vi "11_LAYOUT_COVID_19_KIT.vi"() -> ()   [LabVIEW 2019]
panel:
  in  "INT_TAB":bool
  in  "Tab Control":enum32{"Page 1", "Page 2"}(tab)
  in  "vi path":path
  in  "stop":bool
  # "LAYOUT --> TAB/SUB"
  # "SELECTOR TAB"
  # "(C) 2020"
  # "J.LUIS PÉREZ DEL VAL"
  # "GIF ANIMADO"
  # "KIT o CALENDARIO?..."
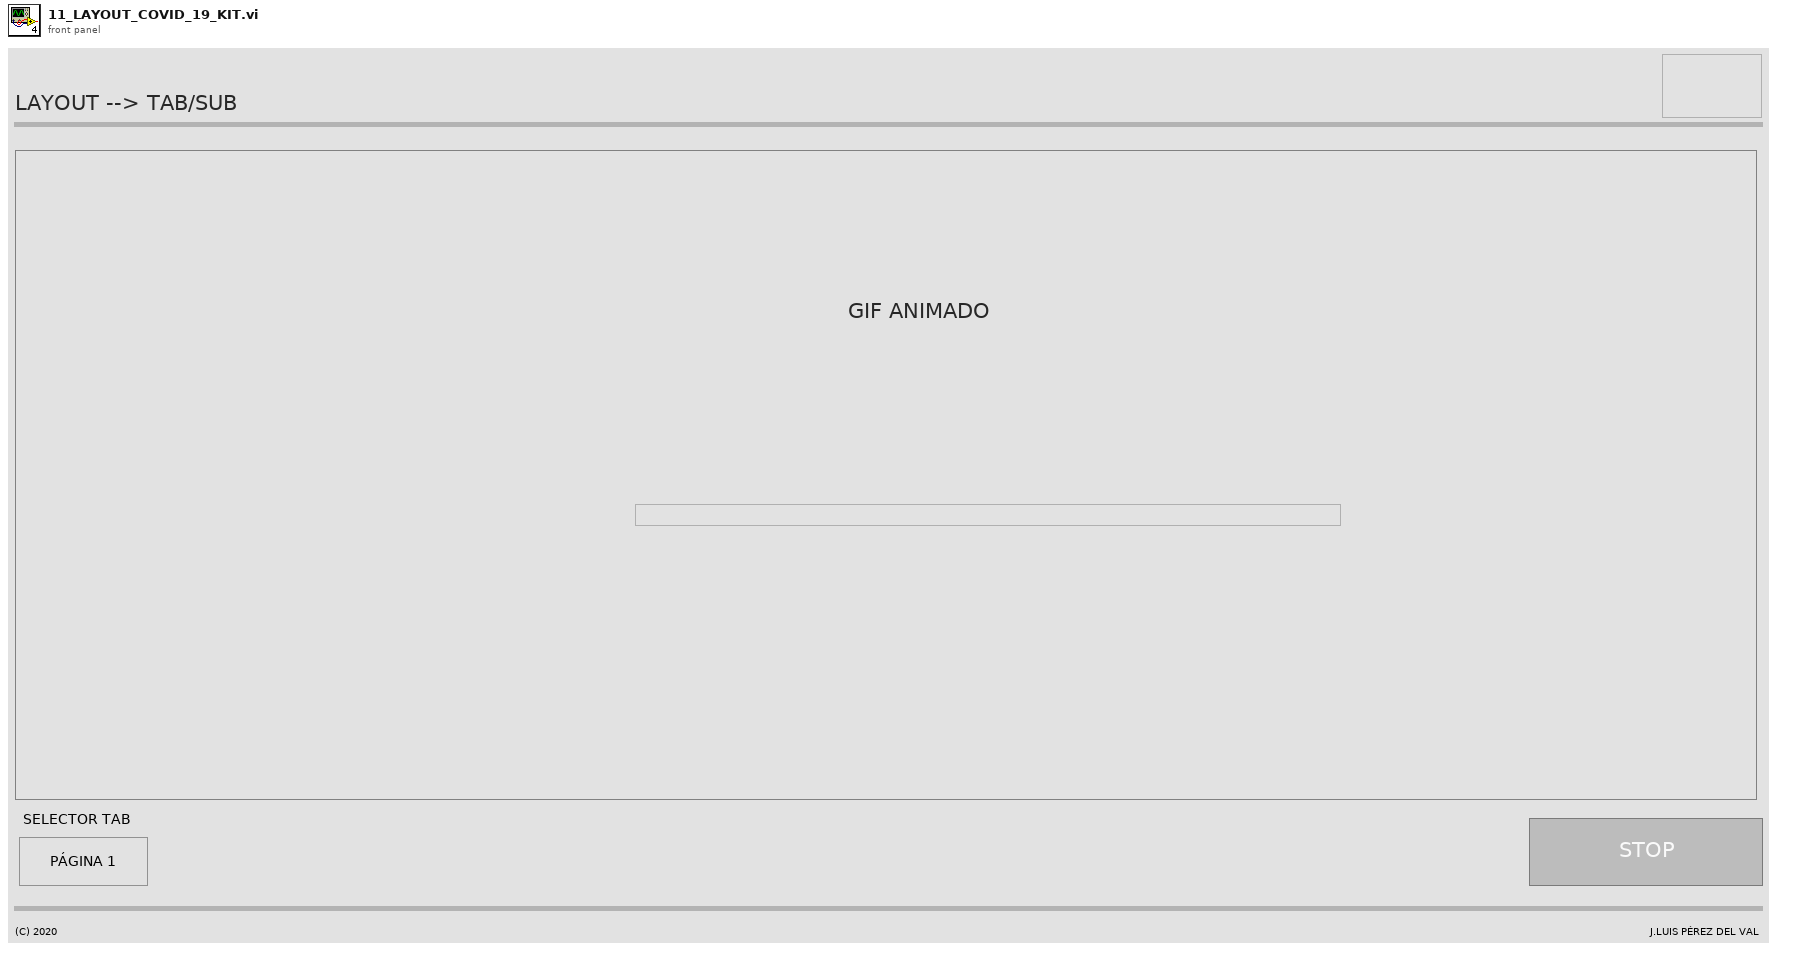
[diagram p1: front panel]
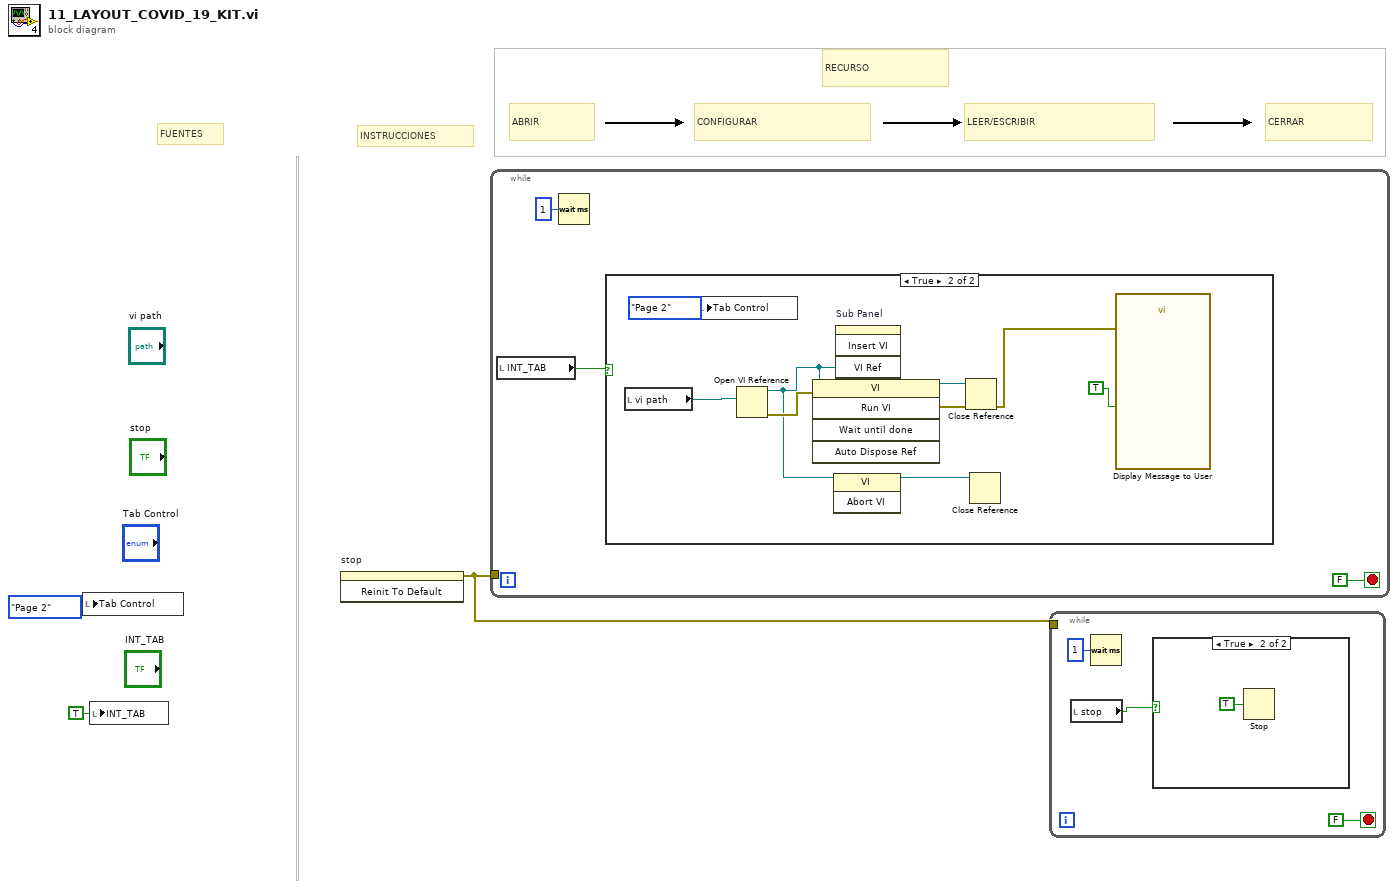
[diagram p0: block diagram]
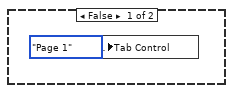
[diagram p3: hidden frame]
diagram:
  # "RECURSO"
  # "CERRAR"
  # "LEER/ESCRIBIR"
  # "CONFIGURAR"
  # "ABRIR"
  # "INSTRUCCIONES"
  # "FUENTES"
  n1 = local write "Tab Control"(enum32{"Page 1", "Page 2"}."Page 2" ("Tab Control 2")) -> ()
  n2 = local write "INT_TAB"(TRUE ("INT_TAB")) -> ()
  n3 = invoke on="stop" class="Bool (strict)" method="Reinit To Default"() -> (error out=w3:errorcluster)  [unwired: 3 in, 2 out]
  n4 = while {
    tunnel: w3 -> [_]
    stop <- FALSE stop-if-true
    n5 = local read "INT_TAB"() -> (w4:bool)
    n6 = Wait (ms)(milliseconds to wait=u32 1) -> ()  [unwired: 1 out]
    n7 = case shown="True" w4 {
      frame False {
        n8 = local write "Tab Control"(enum32{"Page 1", "Page 2"}."Page 1" ("Tab Control")) -> ()
      }
      frame True {
        n9 = local read "vi path"() -> (w16:path)
        n10 = local write "Tab Control"(enum32{"Page 1", "Page 2"}."Page 2" ("Tab Control")) -> ()
        n11 = Open VI Reference(vi path=w16) -> (vi reference=w10:refnum<vi>, error out=w14:errorcluster)  [unwired: 5 in]
        n12 = invoke class="VI" method="Run VI"(reference=w10, error in=w14) -> (reference out=w9:refnum<vi>, error out=w13:errorcluster)  [unwired: 3 in, 3 out]
        n13 = invoke class="VI" method="Abort VI"(reference=w10) -> (reference out=w8:refnum<vi>)  [unwired: 2 in, 2 out]
        n14 = invoke on="Sub Panel" class="SubPnl" method="Insert VI"("VI Ref"=w10) -> ()  [unwired: 3 in, 4 out]
        n15 = Close Reference(reference=w9, error in (no error)=w13) -> (error out=w12:errorcluster)
        n16 = Close Reference(reference=w8) -> ()  [unwired: 1 in, 1 out]
        n17 = call "Display Message to User"("error in (no error)"=w12, "Enable"=TRUE) -> ()  [unwired: 8 in, 2 out]
      }
    }
  }
  n18 = while {
    tunnel: w3 -> [_]
    stop <- FALSE stop-if-true
    n19 = local read "stop"() -> (w17:bool)
    n20 = Wait (ms)(milliseconds to wait=u32 1) -> ()  [unwired: 1 out]
    n21 = case shown="True" w17 {
      frame False {
      }
      frame True {
        n22 = Stop(stop? (T)=TRUE) -> ()
      }
    }
  }
